vi "W&R(Dont Konw Size).vi"(0 "VISA resource name in":refnum<visa-resource-name>, 5 "写入指令/数据":string, 7 "超时":u32=5000, 11 "error in":errorcluster, 12 "比较校验":string) -> (4 "VISA resource name out":refnum<visa-resource-name>, 6 "读取缓冲区":string, 15 "error out":errorcluster)   [LabVIEW 2020]
uses:
  <vilib>/Instr/_visa.llb/VISA Set IO Buffer Mask.ctl
  <vilib>/Instr/_visa.llb/VISA Flush IO Buffer Mask.ctl
panel:
  in  "中断次数":i32
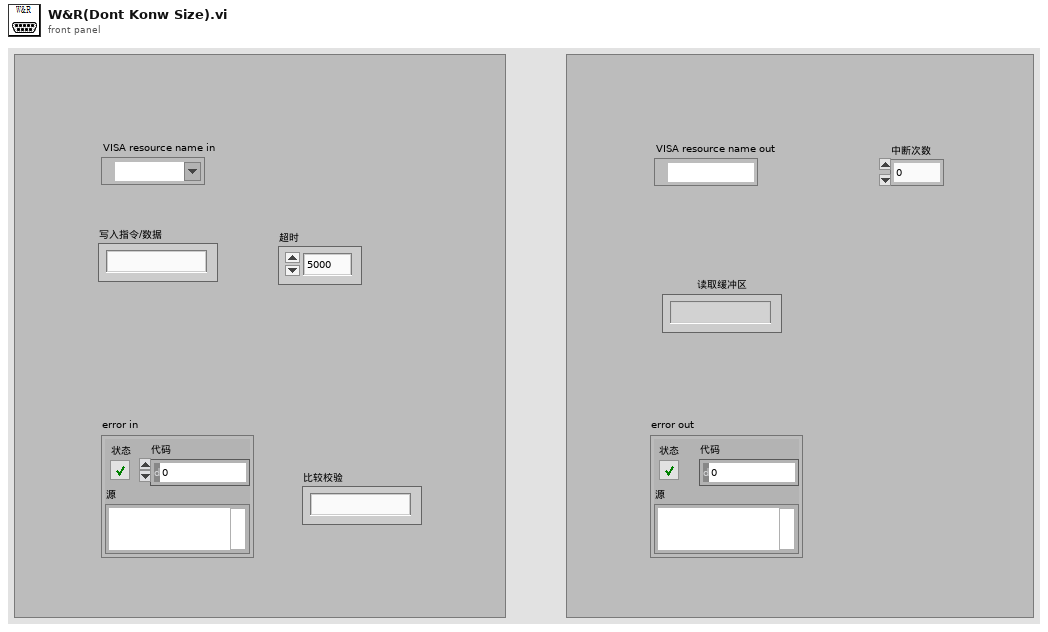
[diagram p1: front panel]
types:
  T1 = typedef "VISA Flush IO Buffer Mask.ctl" = u16
  T2 = typedef "VISA Set IO Buffer Mask.ctl" = u16
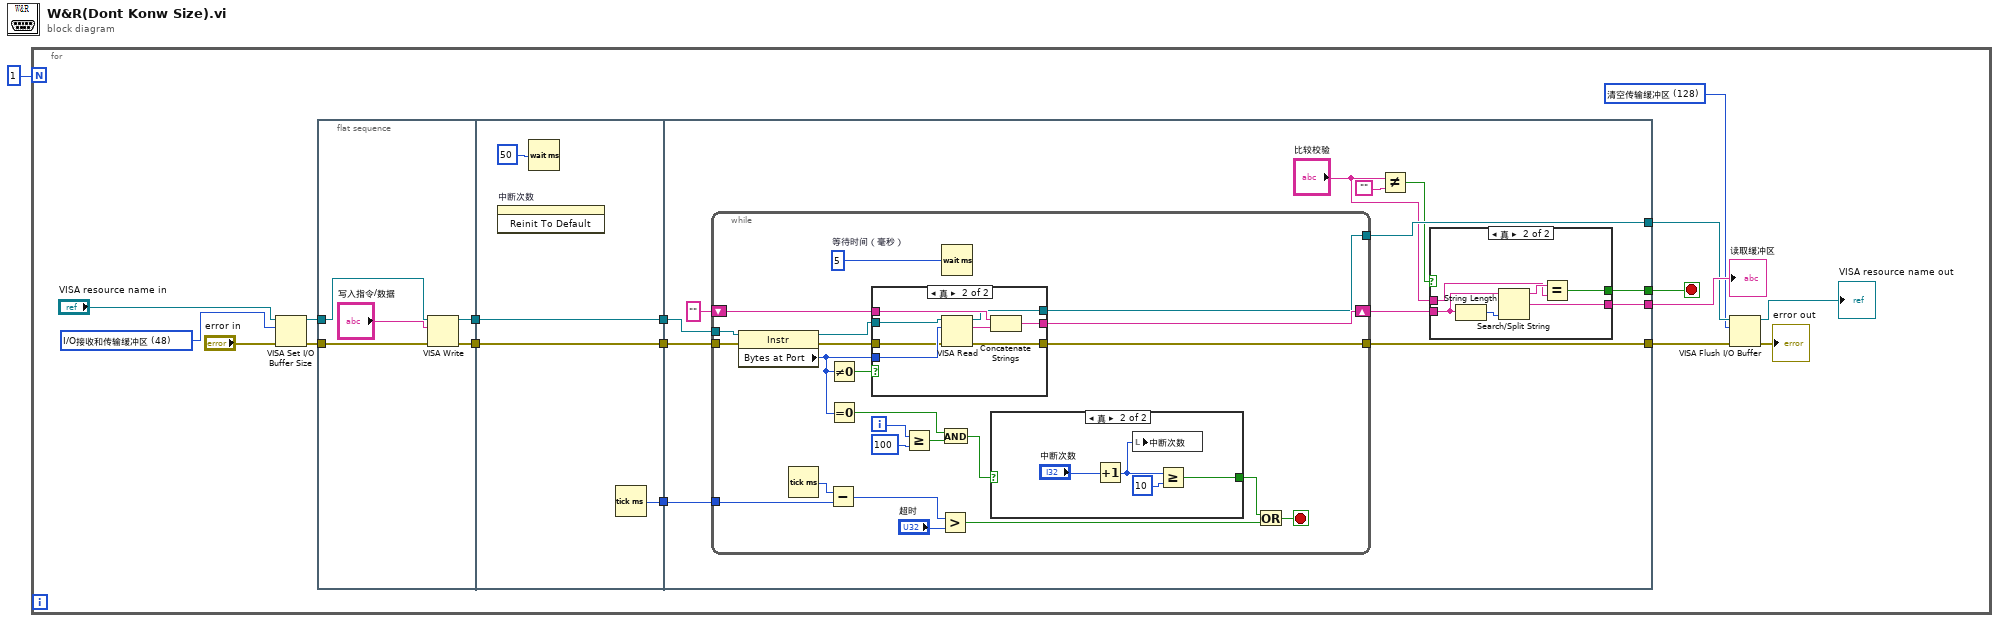
[diagram p0: block diagram]
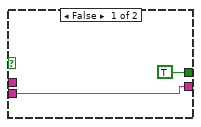
[diagram p2: hidden frame]
diagram:
  n1 = for {
    N: 1 -> [_]
    stop <- w13 stop-if-true
    w2 = T1 128 items=["清空接收缓冲区"=16, "向设备写入传输缓冲区"=32, "清空接收缓冲区（无I/O）"=64, "清空传输缓冲区"=128] ("Mask")
    w7 = T2 48 items=["I/O接收缓冲区"=16, "I/O传输缓冲区"=32, "I/O接收和传输缓冲区"=48] ("Mask")
    n2 = VISA Set I/O Buffer Size(VISA resource name="VISA resource name in", mask (16)=w7, error in (no error)="error in") -> (VISA resource name out=w10:refnum<visa-resource-name>, error out=w8:errorcluster)  [unwired: 1 in]
    n3 = flat-sequence {
      tunnel: w10 -> [w23]
      tunnel: [w22] -> w18
      tunnel: [w20] -> w17
      tunnel: w8 -> [w19]
      tunnel: [w27] -> w16
      tunnel: w18 -> [w27]
      tunnel: [w26] -> w15
      tunnel: w17 -> [w26]
      tunnel: [w25] -> w12
      tunnel: w16 -> [w38]
      tunnel: w15 -> [w37]
      tunnel: [w35] -> w13
      tunnel: [w34] -> w14
      tunnel: [w33] -> w6
      tunnel: [w32] -> w4
      tunnel: w12 -> [w28]
      frame #0 {
        n4 = VISA Write(VISA resource name=w23, write buffer="写入指令/数据", error in (no error)=w19) -> (VISA resource name out=w22:refnum<visa-resource-name>, error out=w20:errorcluster)  [unwired: 1 out]
      }
      frame #1 {
        n5 = invoke on="中断次数" class="DigNum (严格)" method="Reinit To Default"() -> ()  [unwired: 3 in, 3 out]
        n6 = Wait (ms)(milliseconds to wait=u32 50 ("等待时间（毫秒）")) -> ()  [unwired: 1 out]
        n7 = Tick Count (ms)() -> (millisecond timer value=w25:u32)
      }
      frame #2 {
        n8 = while {
          tunnel: w38 -> [w70]
          tunnel: w37 -> [w69]
          shift-right: [w65] -> w36
          shift-left: "" -> [w64]
          tunnel: [w59] -> w33
          tunnel: [w58] -> w32
          tunnel: w28 -> [w49]
          i -> [w57]
          stop <- w61 stop-if-true
          w50 = u32 5  # 等待时间（毫秒）
          n9 = property class="Instr"(reference=w70, error in=w69) -> (reference out=w67:refnum<visa-resource-name>, error out=w66:errorcluster, "Bytes at Port"=w55:u32)
          n10 = Tick Count (ms)() -> (millisecond timer value=w60:u32)
          n11 = Subtract(x=w60, y=w49) -> (x-y=w63:u32)
          n12 = Not Equal To 0?(x=w55) -> (x != 0?=w68:bool)
          n13 = Equal To 0?(x=w55) -> (x = 0?=w54:bool)
          n14 = case shown="真" w68 {
            tunnel: w55 -> [_ w86]
            tunnel: w67 -> [w77 w85]
            tunnel: w66 -> [w76 w84]
            tunnel: [w78 w82] -> w65
            tunnel: w64 -> [w78 w81]
            tunnel: [w77 w80] -> w59
            tunnel: [w76 w79] -> w58
            frame False {
            }
            frame True {
              n15 = VISA Read(VISA resource name=w85, byte count=w86, error in (no error)=w84) -> (VISA resource name out=w80:refnum<visa-resource-name>, read buffer=w83:string, error out=w79:errorcluster)  [unwired: 1 out]
              n16 = Concatenate Strings(w81, w83) -> (w82:string)
            }
          }
          n17 = Greater Or Equal?(x=w57, y=100) -> (x >= y?=w53:bool)
          n18 = Greater?(x=w63, y="超时") -> (0:w62:bool)
          n19 = And(x=w54, y=w53) -> (x .and. y?=w52:bool)
          n20 = Wait (ms)(milliseconds to wait=w50) -> ()  [unwired: 1 out]
          n21 = case shown="真" w52 {
            selector: w52 -> [w71 _]
            tunnel: [w71 w73] -> w51
            frame False {
            }
            frame True {
              n22 = Increment(x="中断次数") -> (x+1=w72:i32)
              n23 = local write "中断次数"(w72) -> ()
              n24 = Greater Or Equal?(x=w72, y=10) -> (x >= y?=w73:bool)
            }
          }
          n25 = Or(x=w51, y=w62) -> (x .or. y?=w61:bool)
        }
        n26 = Not Equal?(x="比较校验", y="") -> (x != y?=w29:bool)
        n27 = case shown="真" w29 {
          tunnel: w36 -> [w41 w43]
          tunnel: [w41 w45] -> w34
          tunnel: [TRUE w46] -> w35
          tunnel: "比较校验" -> [_ w44]
          frame False {
          }
          frame True {
            n28 = String Length(string=w43) -> (length=w42:i32)
            n29 = Search/Split String(string=w43, offset (0)=w42) -> (substring before match=w47:string, match + rest of string=w45:string)  [unwired: 1 in, 1 out]
            n30 = Equal?(x=w47, y=w44) -> (x = y?=w46:bool)
          }
        }
      }
    }
    n31 = VISA Flush I/O Buffer(VISA resource name=w6, mask (16)=w2, error in (no error)=w4) -> (VISA resource name out=→"VISA resource name out":refnum<visa-resource-name>, error out=→"error out":errorcluster)
    "读取缓冲区" <- w14
  }
